vi "Error Msg.vi"(8 "error in (no error)":errorcluster, 11 "[V] Login in":refnum<class "[V] Login.lvclass">) -> (0 "error out":errorcluster, 3 "[V] Login out":refnum<class "[V] Login.lvclass">)   [LabVIEW 2020, in "[V] Login.lvlib" / "[V] Login.lvclass"]
uses:
  [V] Login.lvclass
  [V] Login.lvclass/[V] Login.ctl
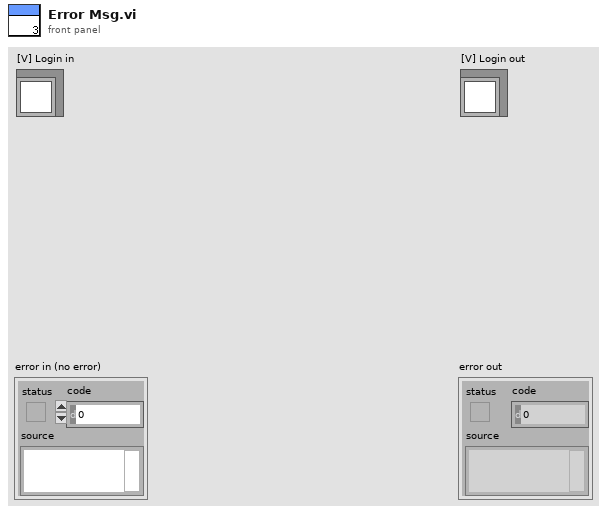
[diagram p1: front panel]
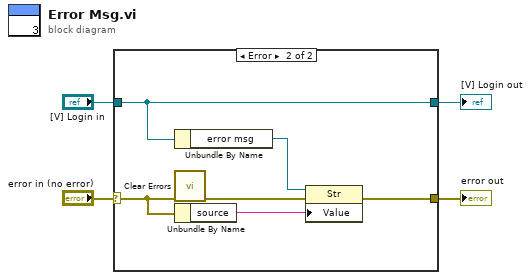
[diagram p0: block diagram]
diagram:
  n1 = case shown="Error" "error in (no error)" {
    selector: "error in (no error)" -> [w5 w9]
    tunnel: [w5 w7] -> w3
    tunnel: [w6 w12] -> w1
    tunnel: "[V] Login in" -> [w6 w12]
    frame No Error {
    }
    frame Error {
      n2 = Unbundle By Name(w12) -> ("error msg"=w10:refnum<vi>)
      n3 = call <vilib>:"Clear Errors.vi"("error in (no error)"=w9) -> ("error out"=w11:errorcluster)  [unwired: 5 in, 1 out]
      n4 = Unbundle By Name(w9) -> ("source"=w8:string)
      n5 = property class="Str"(reference=w10, error in=w11, "Value"=w8) -> (error out=w7:errorcluster)  [unwired: 1 out]
    }
  }
  "error out" <- w3
  "[V] Login out" <- w1
